vi "Diagnostics Response.vi"(8 "error in (no error)":errorcluster, 10 "Modbus Library.lvlib:Modbus Data Unit":refnum<class "Modbus Data Unit.lvclass">) -> (0 "error out":errorcluster, 2 "Data":u16[](array[numeric]))   [LabVIEW 2015, in "Modbus Library.lvlib" / "Master Function Definition.lvclass"]
uses:
  Master Function Definition.lvclass
  Modbus Data Unit/Modbus Data Unit.lvclass
  Modbus Library.lvlib
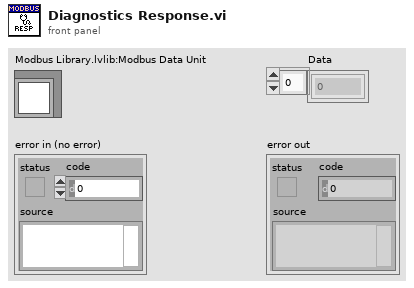
[diagram p1: front panel]
types:
  T1 = typedef "Modbus Library.lvlib/Function.ctl" = u8
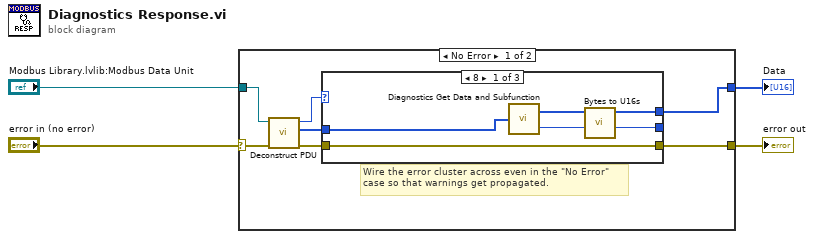
[diagram p0: block diagram]
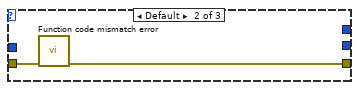
[diagram p2: hidden frame]
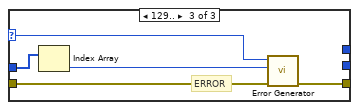
[diagram p3: hidden frame]
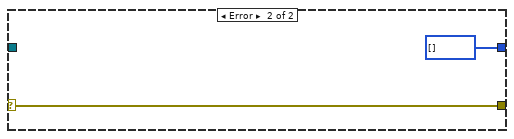
[diagram p4: hidden frame]
diagram:
  n1 = case shown="No Error" "error in (no error)" {
    selector: "error in (no error)" -> [w6 w25]
    tunnel: [w11 w25] -> w3
    tunnel: "Modbus Library.lvlib:Modbus Data Unit" -> [w9 _]
    tunnel: [w10 u16[] [] ("Registers")] -> w2
    frame No Error {
      # "Wire the error cluster across even in the \"No Error\"\ncase so that warnings get propagated."
      n2 = call "Deconstruct PDU.vi"("error in"=w6, "modbus data unit in"=w9) -> ("error out"=w5:errorcluster, "data"=w7:u8[], "Function"=w8:T1)  [unwired: 7 in]
      n3 = case shown="8" w8 {
        selector: w8 -> [_ _ w22]
        tunnel: w5 -> [w13 w18 w20]
        tunnel: w7 -> [w15 _ w23]
        tunnel: [w13 w17 w19] -> w11
        tunnel: [w16 _ _] -> w10
        tunnel: [w12 _ _] -> _
        frame 8 {
          n4 = call "Diagnostics Get Data and Subfunction.vi"("data in"=w15) -> ("subfunction"=w12:u16, "data out"=w14:u8[])  [unwired: 2 in]
          n5 = call "Bytes to U16s.vi"("Bytes"=w14) -> ("Registers"=w16:u16[])  [unwired: 10 in]
        }
        frame Default {
          n6 = call "Function code mismatch error.vi"("error in (no error)"=w18) -> ("error out"=w17:errorcluster)  [unwired: 10 in]
        }
        frame 129.. {
          # "ERROR"
          n7 = Index Array(array=w23) -> (element=w21:u8)  [unwired: 1 in]
          n8 = call "Error Generator.vi"("error in"=w20, "data return (error code)"=w21, "function return"=w22) -> ("error out"=w19:errorcluster)  [unwired: 8 in]
        }
      }
    }
    frame Error {
    }
  }
  "error out" <- w3
  "Data" <- w2
